vi "UpdateMDF.vi"(8 "Index":i32, 11 "MDF_In":T1) -> (2 "MDF_Out":T1)   [LabVIEW 2010]
doc: "This VI updates the status control in the MDF cluster"
uses:
  4-High Neurons/MDFArray.ctl
  4-High Neurons/MissionDefinitionFile.ctl
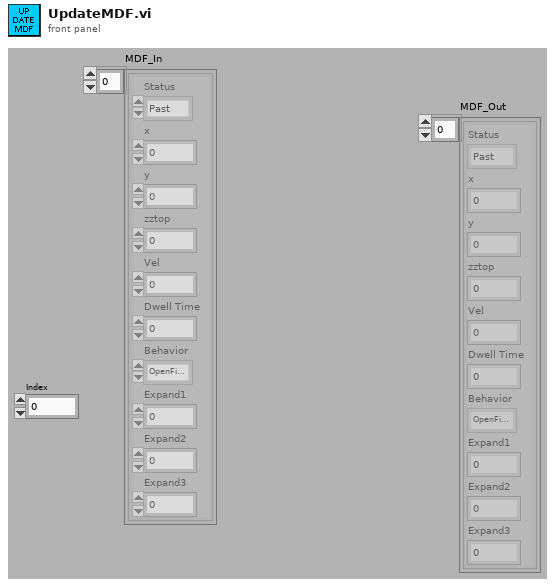
[diagram p1: front panel]
types:
  T1 = typedef "MDFArray.ctl" = T2[]
  T2 = typedef "MissionDefinitionFile.ctl" = cluster{"Status":enum16{"Past", "Current", "Future"}, "x":dbl, "y":dbl, "zztop":dbl, "Vel":dbl, "Dwell Time":dbl, "Behavior":enum16{"OpenFieldTransit", "WallFollow", "LaneFollow", "ManualMode"}, "Expand1":dbl, "Expand2":dbl, "Expand3":dbl}
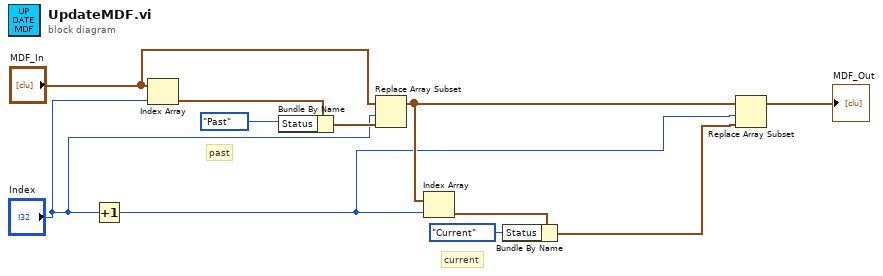
[diagram p0: block diagram]
diagram:
  # "current"
  # "past"
  n1 = Increment(x="Index") -> (x+1=w1:i32)
  n2 = Index Array "Index Array"(array="MDF_In", index="Index") -> (element=w9:T2)
  n3 = Bundle By Name(cluster=w9, "Status"=enum16{"Past", "Current", "Future"}."Past") -> (w8:T2)
  n4 = Replace Array Subset "Replace Array Subset"(array="MDF_In", new element=w8, index="Index") -> (w5:T1)
  n5 = Index Array "Index Array"(array=w5, index=w1) -> (element=w4:T2)
  n6 = Bundle By Name(cluster=w4, "Status"=enum16{"Past", "Current", "Future"}."Current") -> (w2:T2)
  n7 = Replace Array Subset "Replace Array Subset"(array=w5, new element=w2, index=w1) -> (→"MDF_Out":T1)
